vi "config save.vi"(8 "error in (no error)":errorcluster caption="错误输入（无错误）") -> (0 "error out":errorcluster caption="错误输出")   [LabVIEW 2016, in "DR803M4.lvlib"]
uses:
  DR803M4.lvlib
  Global variable/hold variable.vi
  <vilib>/Utility/config.llb/NI_LVConfig.lvlib
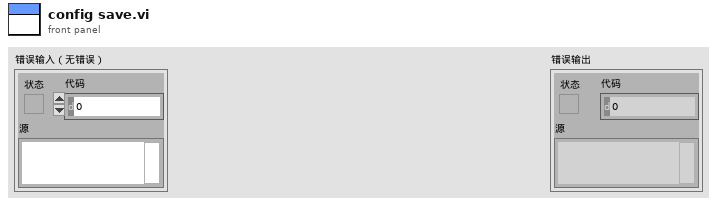
[diagram p1: front panel]
types:
  T1 = typedef "NI_LVConfig.lvlib/Config Data RefNum.ctl" = refnum<k1>
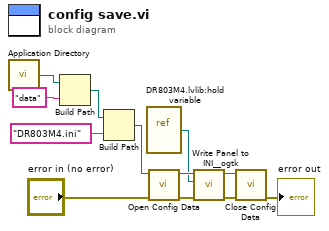
[diagram p0: block diagram]
diagram:
  n1 = call <vilib>:"Application Directory.vi"() -> ("Application Directory"=w8:path)
  n2 = Build Path(base path=w8, name or relative path="data" ("名称或相对路径")) -> (appended path=w6:path)
  n3 = Build Path(base path=w6, name or relative path="DR803M4.ini" ("名称或相对路径")) -> (appended path=w4:path)
  n4 = vi-ref "DR803M4.lvlib:hold variable.vi"() -> (w3:refnum<vi>)
  n5 = call <vilib>:"Open Config Data.vi"("error in (no error)"="error in (no error)", "configuration file path"=w4) -> ("error out"=w11:errorcluster, "refnum"=w12:T1)  [unwired: 7 in, 1 out]
  n6 = call <userlib>:"Write Panel to INI__ogtk.vi"("error in (no error)"=w11, "VI ref"=w3, "refnum"=w12) -> ("error out"=w9:errorcluster, "refnum out"=w10:T1)  [unwired: 7 in]
  n7 = call <vilib>:"Close Config Data.vi"("error in (no error)"=w9, "refnum"=w10) -> ("error out"=→"error out":errorcluster)  [unwired: 8 in, 1 out]
